vi "Log In.vi"(8 "Error In":errorcluster) -> (0 "Error Out":errorcluster, 2 "Password":string, 3 "Username":string)   [LabVIEW 2023, in "Weather Request Loop.lvlib"]
doc: "Prompts the user to enter a username and password in order to log in to the server. The returned client handle may be different from the one input. If this is the case, the old client handle will be closed automatically."
uses:
  Weather Request Loop.lvlib
  <vilib>/Utility/error.llb/Error Cluster From Error Code.vi
  <vilib>/ErrorRing/Error Ring.xnode
panel:
  in  "Cancel Button":bool
  in  "OK Button":bool
  in  "Password Input":string caption="Password"
  in  "Username Input":string caption="Username"
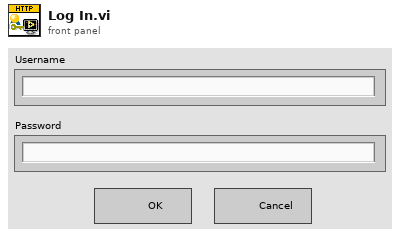
[diagram p1: front panel]
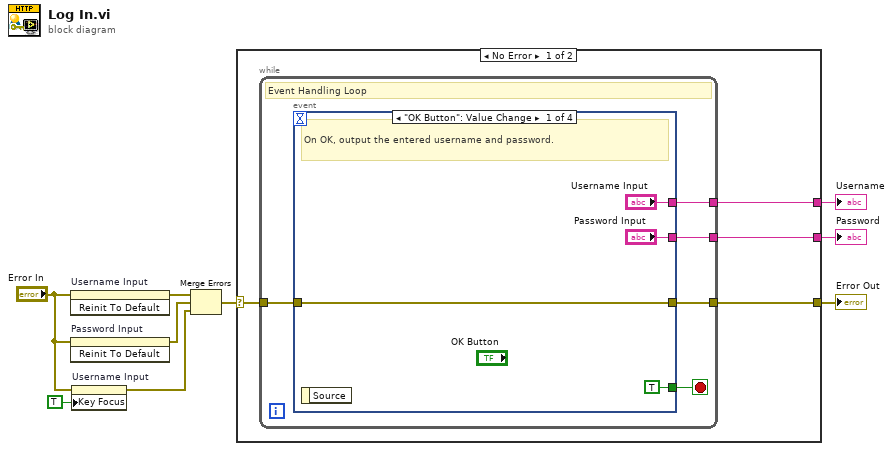
[diagram p0: block diagram]
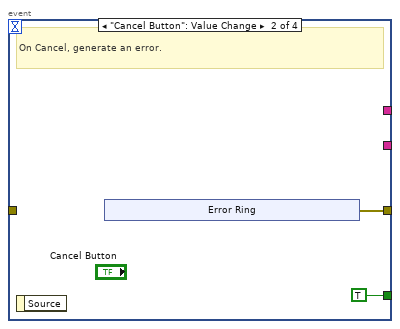
[diagram p2: hidden frame]
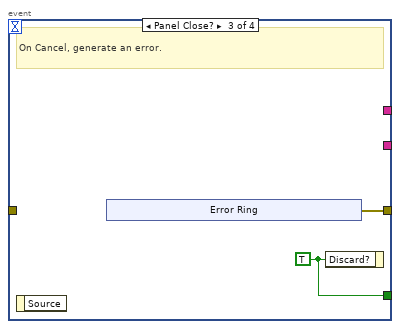
[diagram p3: hidden frame]
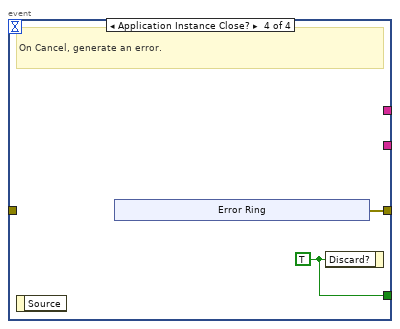
[diagram p4: hidden frame]
diagram:
  n1 = invoke on="Username Input" class="Str" method="Reinit To Default"(error in="Error In") -> (error out=w7:errorcluster)  [unwired: 2 in, 2 out]
  n2 = invoke on="Password Input" class="Str" method="Reinit To Default"(error in="Error In") -> (error out=w5:errorcluster)  [unwired: 2 in, 2 out]
  n3 = property on="Username Input" class="Str"(error in="Error In", "Key Focus"=TRUE) -> (error out=w6:errorcluster)  [unwired: 1 in, 1 out]
  n4 = Merge Errors(w7, w5, w6) -> (w4:errorcluster)
  n5 = case shown="No Error" w4 {
    selector: w4 -> [w13 w41]
    tunnel: [w12 w41] -> w9
    tunnel: [w11 _] -> w2
    tunnel: [w10 _] -> w1
    frame No Error {
      n6 = while {
        tunnel: w13 -> [w17]
        tunnel: [w16] -> w12
        tunnel: [w15] -> w11
        tunnel: [w14] -> w10
        stop <- w18 stop-if-true
        # "Event Handling Loop"
        n7 = event shown="[0] \"OK Button\": Value Change" {
          selector: _ -> [_ _ _ _]
          dyn-events: _ -> [_ _ _ _]
          timeout: _ -> [_ _ _ _]
          tunnel: [TRUE TRUE w30 w36] -> w18
          tunnel: w17 -> [w21 _ _ _]
          tunnel: [w21 w23 w29 w35] -> w16
          tunnel: ["Username Input" _ _ _] -> w15
          tunnel: ["Password Input" _ _ _] -> w14
          event "OK Button": Value Change {
            # "On OK, output the entered username and password."
            n8 = event-data() -> ()  [unwired: 1 in, 1 out]
          }
          event "Cancel Button": Value Change {
            # "On Cancel, generate an error."
            n9 = event-data() -> ()  [unwired: 1 in, 1 out]
            n10 = xnode "Error Ring"() -> ("error out"=w23:errorcluster)
          }
          event Panel Close? {
            w30 = TRUE ("Discard?")
            # "On Cancel, generate an error."
            n11 = event-data() -> ()  [unwired: 1 in, 1 out]
            n12 = xnode "Error Ring"() -> ("error out"=w29:errorcluster)
            n13 = event-data("Discard?"=w30) -> ()  [unwired: 1 in, 1 out]
          }
          event Application Instance Close? {
            w36 = TRUE ("Discard?")
            # "On Cancel, generate an error."
            n14 = event-data() -> ()  [unwired: 1 in, 1 out]
            n15 = xnode "Error Ring"() -> ("error out"=w35:errorcluster)
            n16 = event-data("Discard?"=w36) -> ()  [unwired: 1 in, 1 out]
          }
        }
      }
    }
    frame Error {
    }
  }
  "Error Out" <- w9
  "Username" <- w2
  "Password" <- w1
